vi "ReadImageFileInfo.vi"(8 "error in":errorcluster, 11 "File Path":path) -> (0 "error out":errorcluster, 1 "Height":i32, 2 "Width":i32, 3 "File Type":string, 4 "Image Type":T2, 6 "File Data Type":T1 items=["1 bit", "2 bits", "4 bits", "8 bits", "16 bits (unsigned)", "16 bits (signed)", "16 bits (RGB chunky)", "24 bits (RGB chunky)", "24 bits (RGB planar)", "32 bits (unsigned)", "32 bits (signed)", "32 bits (RGB chunky)", "32 bits (float)", "48 bits (Complex 2x24 int)", "64 bits (Complex 2x32 float)", "32 bits (HSL)"])   [LabVIEW 2024, in "OpenLvVision_Image.lvlib" / "File.lvlib"]
doc: "Returns the information of an save image file"
uses:
  File.lvlib
  Management/TypeDef/ImageType.ctl
  TypeDef/FileDataType.ctl
  Management/Management.lvlib
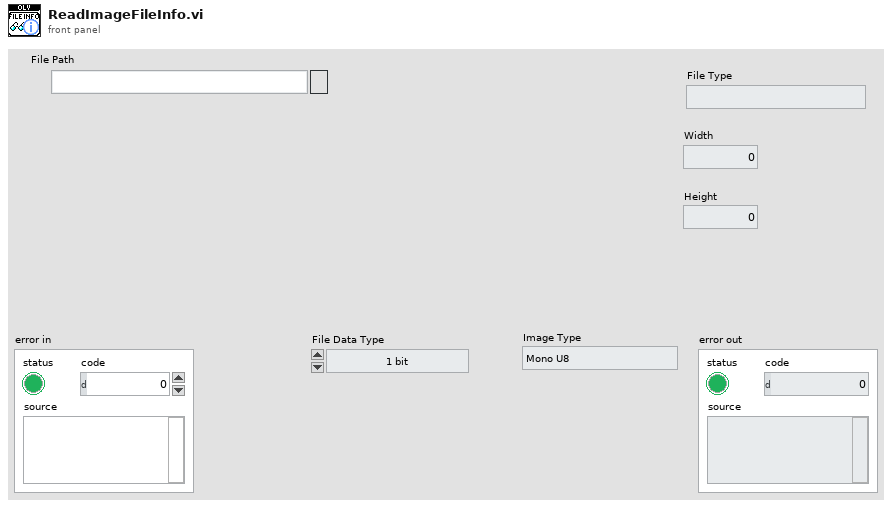
[diagram p1: front panel]
types:
  T1 = typedef "OpenLvVision_Image.lvlib/File.lvlib/FileDataType.ctl" = u32
  T2 = typedef "OpenLvVision_Image.lvlib/Management.lvlib/ImageType.ctl" = enum16{"Mono U8", "Mono U16", "Mono I16", "Mono SGL", "Color U32", "Color U64"}
  T3 = typedef "Image Type" = u32
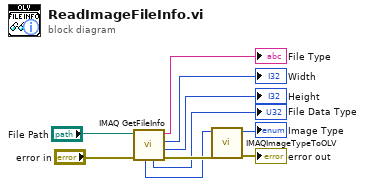
[diagram p0: block diagram]
diagram:
  n1 = call "IMAQ GetFileInfo"("error in (no error)"="error in", "File Path"="File Path") -> ("error out"=w5:errorcluster, "Y Resolution"=→"Height":i32, "X Resolution"=→"Width":i32, "File Type"=→"File Type":string, "File Data Type"=→"File Data Type":i32, "Image Type"=w4:T3)  [unwired: 3 in, 1 out]
  n2 = call "IMAQImageTypeToOLV.vi"("error in"=w5, "IMAQ Image Type"=w4) -> ("error out"=→"error out":errorcluster, "OLV Image Type"=→"Image Type":T2)  [unwired: 8 in]
